vi "Diagnostic.vi"() -> ()   [LabVIEW 2015]
uses:
  Type/_GUI Method.ctl
  Type/_Lens Property.ctl
  Type/_Mass Range Property.ctl
  Type/_Mass Range Parameters.ctl
  Type/_RT Res Type.ctl
  Type/_Run Mode.ctl
  Type/_Run State.ctl
  Type/_File Type.ctl
  Type/_RT Command.ctl
  Type/_Data Operation.ctl
  Type/_Run Module.ctl
  Configuration/_Global Configuration.vi
  <vilib>/Utility/config.llb/Read Key (Path).vi
  <vilib>/Utility/config.llb/Read Key (String).vi
  <vilib>/printing/ReportDocExtensions.llb/Append Front Panel Image to Report (path).vi
  <vilib>/Utility/config.llb/Write Key (Path).vi
  <vilib>/Utility/config.llb/Write Key (String).vi
  <vilib>/Utility/miscctls.llb/LVRectTypeDef.ctl
  <vilib>/Utility/NIReport.llb/NI_report.lvclass
  <vilib>/Utility/NIReport.llb/NI_ReportGenerationCore.lvlib
  <vilib>/Utility/config.llb/NI_LVConfig.lvlib
panel:
  in  "Control 4":bool
  in  "Control 3":bool
  in  "Control 2":bool
  in  "Control 1":bool
  out "H Current 4":dbl
  out "H Current 3":dbl
  out "H Current 2":dbl
  out "H Current 1":dbl
  in  "Heater 4":dbl
  in  "Heater 3":dbl
  in  "Heater 2":dbl
  in  "Heater 1":dbl
  in  "Run Mode":T1
  in  "Q2DC EN":bool
  in  "Count1":dbl=400.0 caption="Lens Value" format="%#.3f"
  in  "Count2":dbl=400.0 caption="High Value" format="%#.3f"
  in  "Time1":dbl=1.0 caption="Low Dwell (ms)" format="%#.3f"
  in  "Time2":dbl=1.0 caption="High Dwell (ms)" format="%#.3f"
  in  "Scans":i32=1
  in  "Step Size":dbl=-1.0 format="%#.3f"
  in  "Scan Type":u8(ring) items=["Single", "Dual", "Ramp"]
  in  "Unit":bool
  in  "Q1DC EN":bool
  in  "Q1 POL":bool
  in  "Q2 POL":bool
  out "DAC Value":i32=98187
  in  "Lens Table":i32(listbox)
  in  "Swtich Polarity":bool
  in  "Run":bool
  out "Dual Run":bool
  out "Spectrum":cluster{"Mass":dbl[], "Data in cps":dbl[]}[](graph)=[{"Mass"=[664.0], "Data in cps"=[]}, {"Mass"=[800.0], "Data in cps"=[]}, {"Mass"=[700.0], "Data in cps"=[]}]
  in  "Cancel":bool
  in  "NewMethod":bool
  in  "Method Path":path
  in  "Method":T2={"Lenses"=[{"Scan Type"=0, "Scans"=1, "Time 1"=1.0, "Time 2"=1.0, "Value 1"=400.0, "Value 2"=400.0, "Step Size"=-1.0}, {"Scan Type"=0, "Scans"=1, "Time 1"=1.0, "Time 2"=1.0, "Value 1"=150.0, "Value 2"=150.0, "Step Size"=1.0}, {"Scan Type"=0, "Scans"=1, "Time 1"=1.0, "Time 2"=1.0, "Value 1"=32000.0, "Value 2"=32000.0, "Step Size"=1.0}, {"Scan Type"=0, "Scans"=1, "Time 1"=1.0, "Time 2"=1.0, "Value 1"=400.0, "Value 2"=400.0, "Step Size"=1.0}, {"Scan Type"=0, "Scans"=1, "Time 1"=1.0, "Time 2"=1.0, "Value 1"=150.0, "Value 2"=150.0, "Step Size"=1.0}, {"Scan Type"=0, "Scans"=1, "Time 1"=1.0, "Time 2"=1.0, "Value 1"=64000.0, "Value 2"=64000.0, "Step Size"=1.0}, {"Scan Type"=0, "Scans"=1, "Time 1"=1.0, "Time 2"=1.0, "Value 1"=420.0, "Value 2"=420.0, "Step Size"=1.0}, {"Scan Type"=0, "Scans"=1, "Time 1"=1.0, "Time 2"=1.0, "Value 1"=30.0, "Value 2"=30.0, "Step Size"=1.0}, {"Scan Type"=0, "Scans"=1, "Time 1"=1.0, "Time 2"=1.0, "Value 1"=15.0, "Value 2"=15.0, "Step Size"=1.0}, {"Scan Type"=0, "Scans"=1, "Time 1"=1.0, "Time 2"=1.0, "Value 1"=0.0, "Value 2"=0.0, "Step Size"=1.0}, {"Scan Type"=0, "Scans"=1, "Time 1"=1.0, "Time 2"=1.0, "Value 1"=0.0, "Value 2"=0.0, "Step Size"=1.0}, {"Scan Type"=0, "Scans"=1, "Time 1"=1.0, "Time 2"=1.0, "Value 1"=0.0, "Value 2"=0.0, "Step Size"=1.0}, {"Scan Type"=0, "Scans"=1, "Time 1"=1.0, "Time 2"=1.0, "Value 1"=0.0, "Value 2"=0.0, "Step Size"=1.0}, {"Scan Type"=0, "Scans"=1, "Time 1"=1.0, "Time 2"=1.0, "Value 1"=0.0, "Value 2"=0.0, "Step Size"=1.0}, {"Scan Type"=0, "Scans"=1, "Time 1"=1.0, "Time 2"=1.0, "Value 1"=-0.5, "Value 2"=-0.5, "Step Size"=1.0}, {"Scan Type"=0, "Scans"=1, "Time 1"=1.0, "Time 2"=1.0, "Value 1"=-2.0, "Value 2"=-2.0, "Step Size"=1.0}, {"Scan Type"=0, "Scans"=1, "Time 1"=1.0, "Time 2"=1.0, "Value 1"=-1.2, "Value 2"=-1.2, "Step Size"=1.0}, {"Scan Type"=0, "Scans"=1, "Time 1"=1.0, "Time 2"=1.0, "Value 1"=0.0, "Value 2"=0.0, "Step Size"=1.0}, {"Scan Type"=0, "Scans"=1, "Time 1"=1.0, "Time 2"=1.0, "Value 1"=-240.0, "Value 2"=-240.0, "Step Size"=1.0}, {"Scan Type"=0, "Scans"=1, "Time 1"=1.0, "Time 2"=1.0, "Value 1"=-50.0, "Value 2"=-50.0, "Step Size"=1.0}, {"Scan Type"=0, "Scans"=1, "Time 1"=1.0, "Time 2"=1.0, "Value 1"=-52.0, "Value 2"=-52.0, "Step Size"=1.0}, {"Scan Type"=0, "Scans"=1, "Time 1"=1.0, "Time 2"=1.0, "Value 1"=-100.0, "Value 2"=-100.0, "Step Size"=1.0}, {"Scan Type"=0, "Scans"=1, "Time 1"=1.0, "Time 2"=1.0, "Value 1"=-54.0, "Value 2"=-54.0, "Step Size"=1.0}, {"Scan Type"=0, "Scans"=1, "Time 1"=1.0, "Time 2"=1.0, "Value 1"=-400.0, "Value 2"=-400.0, "Step Size"=1.0}, {"Scan Type"=0, "Scans"=1, "Time 1"=1.0, "Time 2"=1.0, "Value 1"=30.0, "Value 2"=30.0, "Step Size"=1.0}, {"Scan Type"=0, "Scans"=1, "Time 1"=1.0, "Time 2"=1.0, "Value 1"=2000.0, "Value 2"=2000.0, "Step Size"=1.0}, {"Scan Type"=0, "Scans"=1, "Time 1"=1.0, "Time 2"=1.0, "Value 1"=-6000.0, "Value 2"=-6000.0, "Step Size"=1.0}, {"Scan Type"=0, "Scans"=1, "Time 1"=1.0, "Time 2"=1.0, "Value 1"=0.0, "Value 2"=0.0, "Step Size"=1.0}, {"Scan Type"=0, "Scans"=1, "Time 1"=1.0, "Time 2"=1.0, "Value 1"=0.0, "Value 2"=0.0, "Step Size"=1.0}, {"Scan Type"=0, "Scans"=1, "Time 1"=1.0, "Time 2"=1.0, "Value 1"=250.0, "Value 2"=250.0, "Step Size"=1.0}, {"Scan Type"=0, "Scans"=1, "Time 1"=1.0, "Time 2"=1.0, "Value 1"=-250.0, "Value 2"=-250.0, "Step Size"=1.0}, {"Scan Type"=0, "Scans"=1, "Time 1"=1.0, "Time 2"=1.0, "Value 1"=250.0, "Value 2"=250.0, "Step Size"=1.0}, {"Scan Type"=0, "Scans"=1, "Time 1"=1.0, "Time 2"=1.0, "Value 1"=-250.0, "Value 2"=-250.0, "Step Size"=1.0}, {"Scan Type"=0, "Scans"=1, "Time 1"=1.0, "Time 2"=1.0, "Value 1"=500.0, "Value 2"=500.0, "Step Size"=1.0}, {"Scan Type"=0, "Scans"=1, "Time 1"=1.0, "Time 2"=1.0, "Value 1"=-500.0, "Value 2"=-500.0, "Step Size"=1.0}, {"Scan Type"=0, "Scans"=1, "Time 1"=1.0, "Time 2"=1.0, "Value 1"=0.55, "Value 2"=0.55, "Step Size"=1.0}, {"Scan Type"=0, "Scans"=1, "Time 1"=1.0, "Time 2"=1.0, "Value 1"=0.0, "Value 2"=0.0, "Step Size"=1.0}, {"Scan Type"=0, "Scans"=1, "Time 1"=1.0, "Time 2"=1.0, "Value 1"=100.0, "Value 2"=100.0, "Step Size"=1.0}, {"Scan Type"=0, "Scans"=1, "Time 1"=1.0, "Time 2"=1.0, "Value 1"=0.0, "Value 2"=0.0, "Step Size"=1.0}, {"Scan Type"=0, "Scans"=1, "Time 1"=1.0, "Time 2"=1.0, "Value 1"=5.0, "Value 2"=5.0, "Step Size"=1.0}, {"Scan Type"=0, "Scans"=1, "Time 1"=1.0, "Time 2"=1.0, "Value 1"=0.0, "Value 2"=0.0, "Step Size"=1.0}, {"Scan Type"=0, "Scans"=1, "Time 1"=1.0, "Time 2"=1.0, "Value 1"=0.0, "Value 2"=0.0, "Step Size"=1.0}, {"Scan Type"=0, "Scans"=1, "Time 1"=1.0, "Time 2"=1.0, "Value 1"=100.0, "Value 2"=100.0, "Step Size"=1.0}, {"Scan Type"=0, "Scans"=1, "Time 1"=1.0, "Time 2"=1.0, "Value 1"=0.0, "Value 2"=0.0, "Step Size"=1.0}, {"Scan Type"=0, "Scans"=1, "Time 1"=1.0, "Time 2"=1.0, "Value 1"=5.0, "Value 2"=5.0, "Step Size"=1.0}, {"Scan Type"=0, "Scans"=1, "Time 1"=1.0, "Time 2"=1.0, "Value 1"=5000.0, "Value 2"=5000.0, "Step Size"=1.0}, {"Scan Type"=0, "Scans"=1, "Time 1"=1.0, "Time 2"=1.0, "Value 1"=0.0, "Value 2"=0.0, "Step Size"=1.0}, {"Scan Type"=0, "Scans"=1, "Time 1"=1.0, "Time 2"=1.0, "Value 1"=100.0, "Value 2"=100.0, "Step Size"=1.0}, {"Scan Type"=0, "Scans"=1, "Time 1"=1.0, "Time 2"=1.0, "Value 1"=0.0, "Value 2"=0.0, "Step Size"=1.0}, {"Scan Type"=0, "Scans"=1, "Time 1"=1.0, "Time 2"=1.0, "Value 1"=5.0, "Value 2"=5.0, "Step Size"=1.0}, {"Scan Type"=0, "Scans"=1, "Time 1"=1.0, "Time 2"=1.0, "Value 1"=1000.0, "Value 2"=1000.0, "Step Size"=1.0}, {"Scan Type"=0, "Scans"=1, "Time 1"=1.0, "Time 2"=1.0, "Value 1"=1.0, "Value 2"=1.0, "Step Size"=1.0}], "Mass Ranges"=[], "Acquire"=FALSE, "MCA"=FALSE, "Q1DC EN"=FALSE, "Q1 POL"=FALSE, "Q3 POL"=FALSE, "Q1 RF  EN"=FALSE, "Averaging"=FALSE, "Log Scale"=FALSE, "CPS"=FALSE, "Unit"=FALSE, "Data Path"=path "", "Run Mode"=enum."MRM (Q1/Q2)", "Fixed Mass (amu)"=0.0, "Q3DC EN"=FALSE, "Q3 RF  EN"=FALSE, "Negative"=FALSE} {"Mass Ranges"."Res" items=["High/High", "Medium/Medium", "Low/Low", "High/Medium", "High/Low", "Medium/High", "Medium/Low", "Low/High", "Low/Medium"]}
  out "Run Time":i32 caption="Run Time (ms)"
  in  "Log Scale":bool
  in  "Scan#":u32=1 caption="Current Scan #"
  in  "CPS":bool
  in  "Averaging":bool
  in  "MCA":bool
  in  "Acquire":bool
  in  "BloUpdate":bool
  out "Data File:":path=path "C:/Users/Min/Projects/Sniffer"
  # "Selected Lens Property"
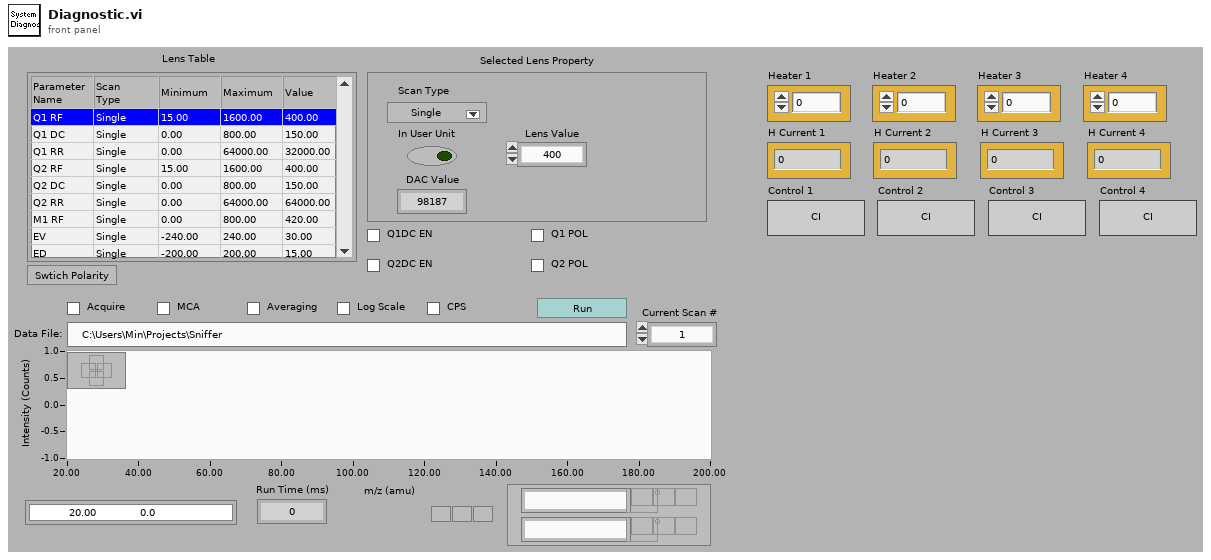
[diagram p1: front panel]
types:
  T1 = typedef "_Run Mode.ctl" = enum16{"MRM (Q1/Q2)", "Q1 Scan", "Q1 SRM", "Q2 Scan", "Q2 SRM", "Product Scan", "Precursor Scan", "Neutral Loss", "Neutral Gain"}
  T2 = typedef "_GUI Method.ctl" = cluster{"Lenses":T3[], "Mass Ranges":T4[], "Acquire":bool, "MCA":bool, "Q1DC EN":bool, "Q1 POL":bool, "Q3 POL":bool, "Q1 RF  EN":bool, "Averaging":bool, "Log Scale":bool, "CPS":bool, "Unit":bool, "Data Path":path, "Run Mode":T1, "Fixed Mass (amu)":dbl, "Q3DC EN":bool, "Q3 RF  EN":bool, "Negative":bool}
  T3 = typedef "_Lens Property.ctl" = cluster{"Scan Type":u8, "Scans":i32, "Time 1":dbl, "Time 2":dbl, "Value 1":dbl, "Value 2":dbl, "Step Size":dbl}
  T4 = typedef "_Mass Range Property.ctl" = cluster{"Start":dbl, "Stop":dbl, "Step Size":dbl, "Steps":i32, "Dwell":dbl, "Parameters":T5[], "Res":T6}
  T5 = typedef "_Mass Range Parameters.ctl" = cluster{"Name":string, "Ch#":u8, "StartV":dbl, "StopV":dbl, "StepV":dbl, "Index":u8}
  T6 = typedef "_RT Res Type.ctl" = u16
  T7 = typedef "_Run State.ctl" = enum16{"Init", "Update", "Start", "End", "Error"}
  T8 = typedef "_RT Instrument 2.ctl" = cluster{"Table":T9[], "Instrument":string[]}
  T9 = typedef "_RT Configuration 2.ctl" = cluster{"Name":string, "Ch#":u8, "Min":dbl, "Max":dbl, "Def+":dbl, "Def-":dbl, "Offset":dbl, "Slope":dbl, "Type":u8, "Description":string, "SettleT":dbl}
  T10 = typedef "_File Type.ctl" = enum16{"Configuration", "Old Configuration", "Calibration", "Resolution", "Diagnostic Method", "Old Method", "Acq Method", "Samp List"}
  T11 = typedef "LVRectTypeDef.ctl" = cluster{"Left":i16, "Top":i16, "Right":i16, "Bottom":i16}
  T12 = enum16{"Standard Report", "HTML", "Word", "Excel"}
  T13 = typedef "_RT Command.ctl" = enum16{"xml Start Run", "xml Start Actual Run", "xml Stop Run", "xml Runtime Update", "xml Get Status", "xml Get Table", "xml Set Table", "xml Get Configuration", "xml System Status", "xml Set LC Input Logic", "xml Get Data", "xml Get Info", "Start", "StartActualRun", "Stop", "Runtime Update", "Get Data", "Get Info", "Get Status", "Get Param", "Get Config", "Get Table", "Read ADC", "Set Oscillator", "Update Config", "Update Table", "Set All Pol", "Set Pol and DC", "Set Max Mass", "Toggle RP", "Toggle EL", "Set PIC", "Initialize Turbo", "Send Turbo Comm", "Close Turbo", "P1", "P2", "P3", "Send Serial", "Set LC Out", "Get LC In", "Read VAC", "Test Table", "Toggle Power", "Get Startup", "Set Startup", "Get ADC Table", "Set ADC Table", "Get Brief Status", "Get Detail Status", "Auxiliary Update", "Set CC Logics", "Set CC Input Logics", "Ignore Error", "invalid"}
  T14 = typedef "_Data Operation.ctl" = enum8{"Initialize", "Get Data", "Set Data", "Close"}
  T15 = enum32{"Bad", "Idle", "Run top level", "Running"}
  T16 = typedef "NI_LVConfig.lvlib/Config Data RefNum.ctl" = refnum<k1>
  T17 = cluster{"Method":T2, "Update":bool, "Running":bool, "Method Path":path}
  T18 = typedef "_Current Data.ctl" = cluster{"Scan#":i32, "Run Time (mS)":i32, "TIC X":dbl[], "TIC Y":dbl[][], "MassRange":cluster{"X Title":string, "X":dbl[], "Y":i32[]}[], "Fixed Mass (amu)":dbl, "Method":T19}
  T19 = typedef "_XML Expt.ctl" = cluster{"StartT(mS)":i32, "#Cycles":i32, "PauseT(uS)":i32, "ScanType":i32, "Polarity":u8, "FixedMass":dbl, "DelayT(mS)":i32, "Active Ch":T20[], "Mass Range":T4[]}
  T20 = typedef "_XML Lens.ctl" = cluster{"Value":dbl, "ChID":u8}
  T21 = cluster{"Scan Type":u8, "Unit":bool, "Count1":dbl, "Count2":dbl, "Time1":dbl, "Time2":dbl, "Scans":i32, "Step Size":dbl, "Lens Table":i32}
  T22 = cluster{"Scan Type":u8, "Unit":bool, "Count1":dbl, "Count2":dbl, "Time1":dbl, "Time2":dbl, "Scans":i32, "Step Size":dbl, "Start DAC":i32, "Ramp Time (ms)":i32}
  T23 = cluster{bool, "Value 1":dbl, "Value 2":dbl, "Step Size":dbl}
  T24 = typedef "_Run Module.ctl" = u16
  T25 = cluster{"NewVal":bool, "Count1":dbl, "Count2":dbl, "Step Size":dbl}
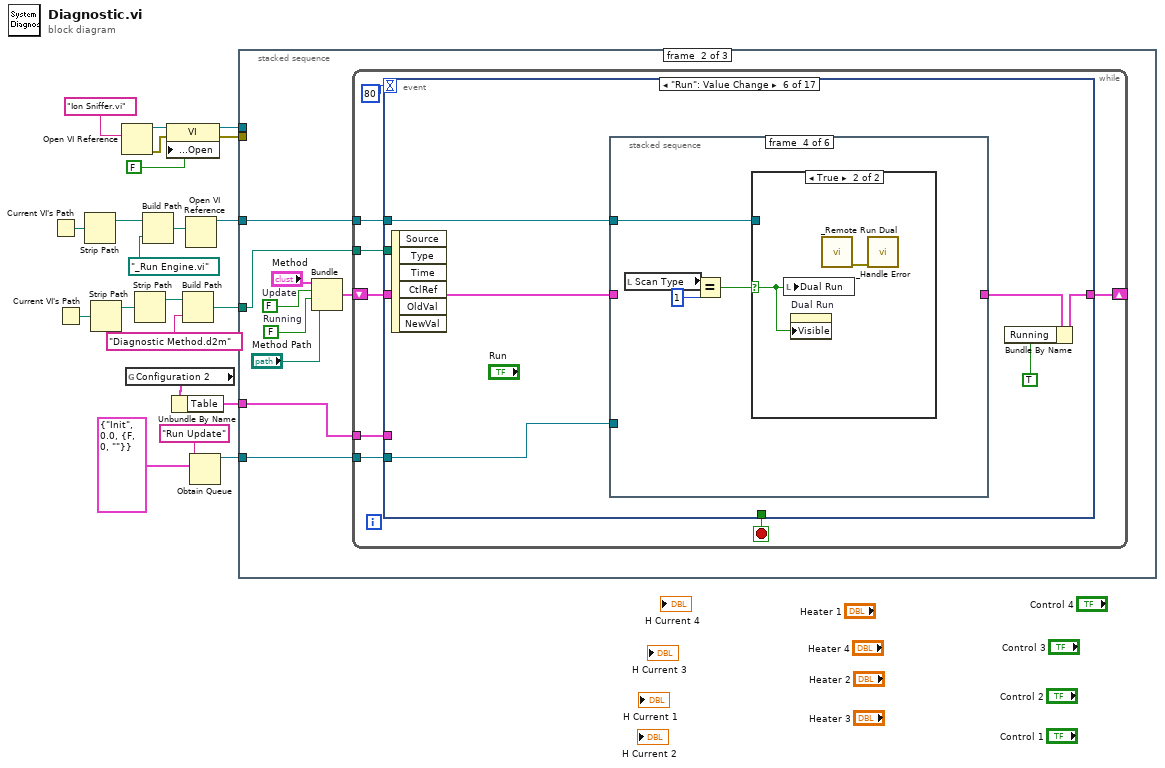
[diagram p0: block diagram]
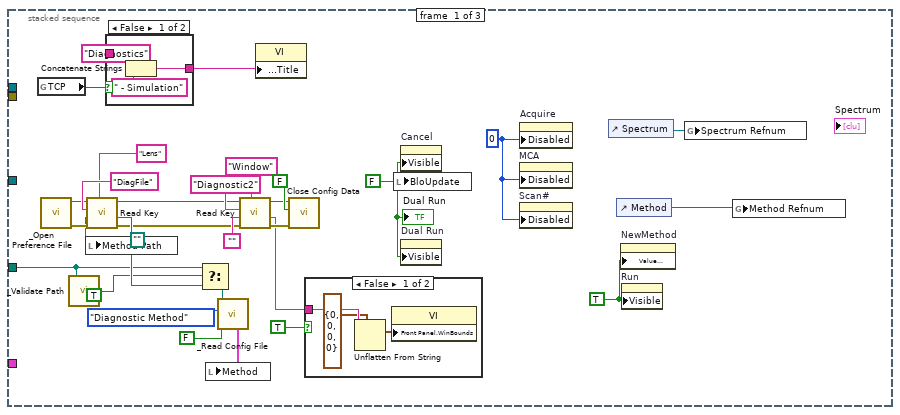
[diagram p2: hidden frame]
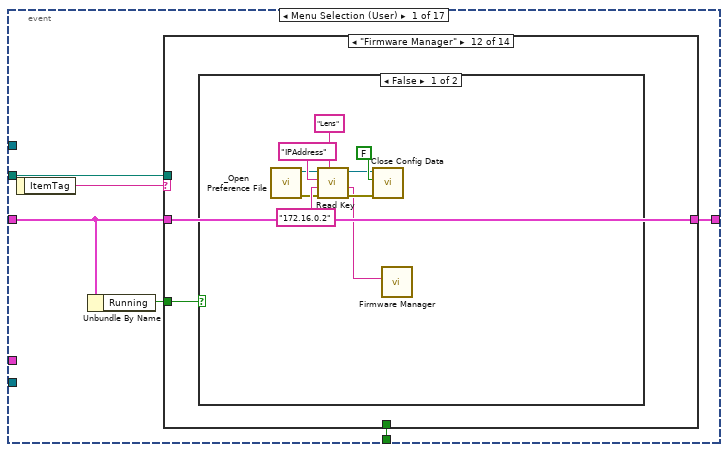
[diagram p5: hidden frame]
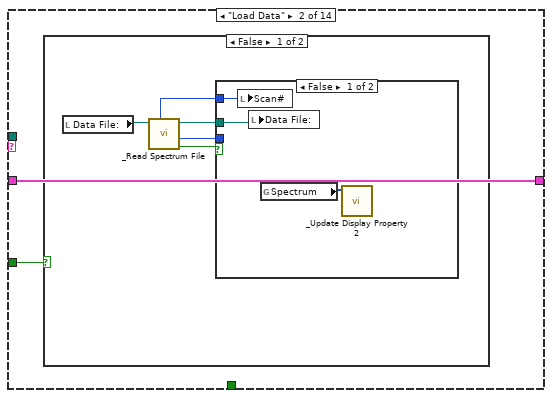
[diagram p7: hidden frame]
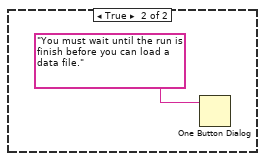
[diagram p9: hidden frame]
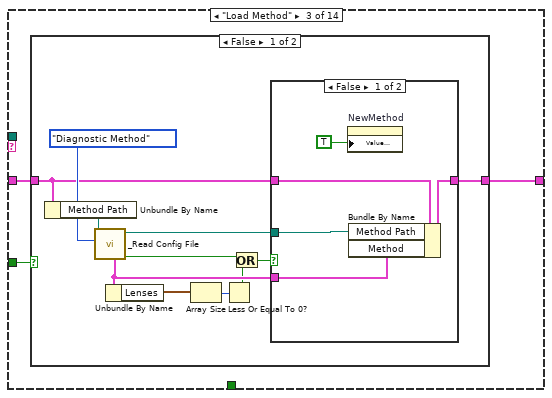
[diagram p10: hidden frame]
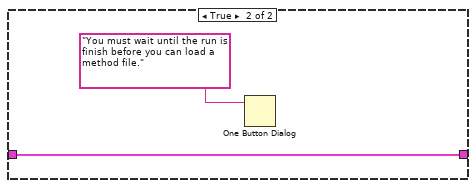
[diagram p12: hidden frame]
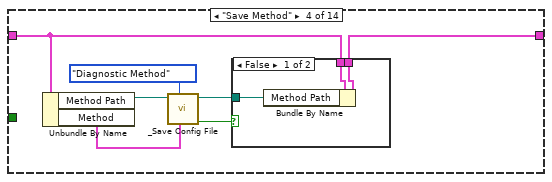
[diagram p13: hidden frame]
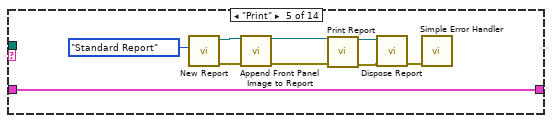
[diagram p15: hidden frame]
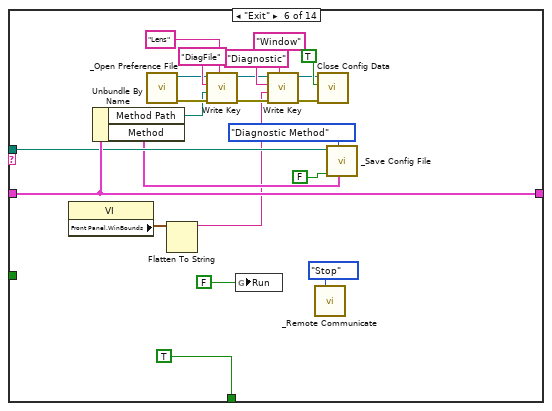
[diagram p16: hidden frame]
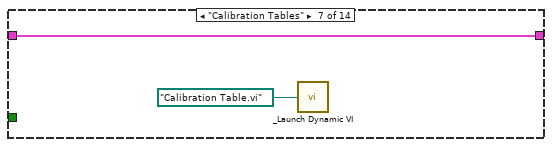
[diagram p17: hidden frame]
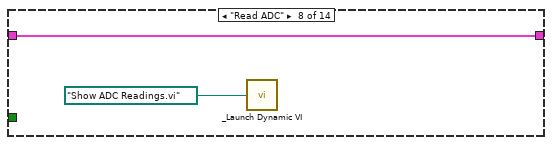
[diagram p18: hidden frame]
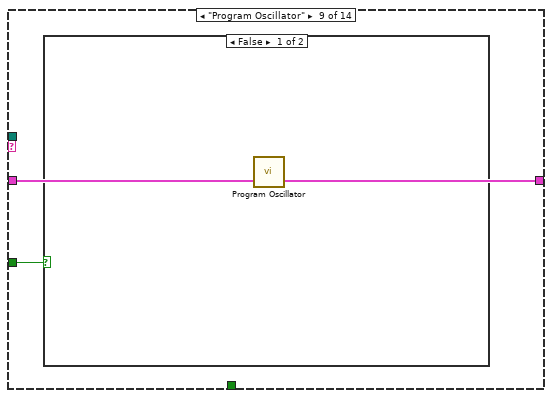
[diagram p19: hidden frame]
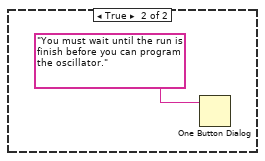
[diagram p20: hidden frame]
diagram:
  n1 = Current VI's Path() -> (path=w18:path)
  n2 = Current VI's Path() -> (path=w8:path)
  n3 = Strip Path(path=w18) -> (stripped path=w14:path)  [unwired: 1 out]
  n4 = Strip Path(path=w8) -> (stripped path=w9:path)  [unwired: 1 out]
  n5 = Open VI Reference(vi path="Ion Sniffer.vi") -> (vi reference=w5:refnum<vi>, error out=w4:errorcluster)  [unwired: 1 in, 4 out]
  n6 = global read "_Global Configuration.vi" "Configuration 2"() -> (w13:T8)
  n7 = Strip Path(path=w9) -> (stripped path=w10:path)  [unwired: 1 out]
  n8 = Build Path(base path=w14, name or relative path=path "_Run Engine.vi") -> (appended path=w16:path)
  n9 = property class="VI"(reference=w5, error in=w4, "Front Panel Window:Open"=FALSE) -> (reference out=w2:refnum<vi>, error out=w1:errorcluster)
  n10 = Unbundle By Name(w13) -> ("Table"=w12:T9[])
  n11 = Build Path(base path=w10, name or relative path="Diagnostic Method.d2m") -> (appended path=w7:path)
  n12 = Open VI Reference(vi path=w16) -> (vi reference=w15:refnum<vi>)  [unwired: 1 in, 5 out]
  n13 = Obtain Queue(name (unnamed)="Run Update", element data type=cluster{T7, dbl, "error out":errorcluster} {enum."Init", 0.0, "error out"={"status"=FALSE, "code"=0, "source"=""}}) -> (queue out=w19:refnum<queue>)  [unwired: 3 in, 2 out]
  n14 = stacked-sequence {
    tunnel: w19 -> [_ w68 w630]
    tunnel: w15 -> [_ w67 w629]
    tunnel: w12 -> [_ w61 _]
    tunnel: w7 -> [w24 w60 _]
    tunnel: w2 -> [_ _ w625]
    tunnel: w1 -> [_ _ w624]
    frame #0 {
      w28 = TRUE ("Visible")
      w49 = u8 0 ("Disabled")
      w42 = FALSE ("Unit")
      n15 = global read "_Global Configuration.vi" "TCP"() -> (w50:bool)
      n16 = call "_Open Preference File.vi"() -> ("error"=w45:errorcluster, "refnum"=w46:T16)  [unwired: 3 in, 3 out]
      n17 = call "_Validate Path.vi"("Check Exist (F)"=TRUE, "path"=w24) -> ("Valid"=w25:bool)  [unwired: 2 in]
      n18 = call-poly <vilib>:"Read Key.vi"("section"="Lens", "error in (no error)"=w45, "default value"=path "", "key"="DiagFile", "refnum"=w46) -> ("error out"=w32:errorcluster, "value"=w38:path, "refnum out"=w33:T16)  [unwired: 4 out]
      n19 = local write "Method Path"(w38) -> ()
      n20 = case shown="False" w50 {
        tunnel: "Diagnostics" ("string") -> [w58 w59]
        tunnel: [w56 w59] -> w51
        frame False {
          n21 = Concatenate Strings(w58, " - Simulation" ("string")) -> (w56:string)
        }
        frame True {
        }
      }
      n22 = Select(t=w24, s=w25, f=w38) -> (s? t:f=w37:path)
      n23 = call "_Read Config File.vi"("advisory dialog? (display:T)"=FALSE, "File Type (config)"=_File_Type."Diagnostic Method", "start path  (Not A Path)"=w37) -> ("GUI Method"=w40:T2)  [unwired: 8 out]
      n24 = local write "Method"(w40) -> ()
      n25 = call-poly <vilib>:"Read Key.vi"("section"="Window", "error in (no error)"=w32, "default value"="", "key"="Diagnostic2" ("section"), "refnum"=w33) -> ("error out"=w30:errorcluster, "value"=w29:string, "refnum out"=w31:T16)  [unwired: 1 in, 3 out]
      n26 = property class="VI"("Front Panel Window:Title"=w51) -> ()  [unwired: 2 in, 2 out]
      n27 = call <vilib>:"Close Config Data.vi"("error in (no error)"=w30, "write file if changed (T)"=FALSE ("write configuration file? (F)"), "refnum"=w31) -> ()  [unwired: 9 out]
      n28 = case shown="False" TRUE {
        tunnel: w29 -> [w55 _]
        frame False {
          n29 = Unflatten From String(type=T11 {"Left"=0, "Top"=0, "Right"=0, "Bottom"=0} ("Front Panel Window:Window Bounds"), binary string=w55) -> (value=w53:T11)  [unwired: 1 in, 4 out]
          n30 = property class="VI"("Front Panel.WinBounds"=w53) -> ()  [unwired: 2 in, 2 out]
        }
        frame True {
        }
      }
      n31 = local write "BloUpdate"(w42) -> ()
      n32 = property on="Cancel" class="Bool"("Visible"=w42) -> ()  [unwired: 2 in, 2 out]
      n33 = property on="Dual Run" class="Bool (strict)"("Visible"=w42) -> ()  [unwired: 2 in, 2 out]
      n34 = property on="Acquire" class="Bool (strict)"("Disabled"=w49) -> ()  [unwired: 2 in, 2 out]
      n35 = property on="MCA" class="Bool (strict)"("Disabled"=w49) -> ()  [unwired: 2 in, 2 out]
      n36 = property on="Scan#" class="DigNum (strict)"("Disabled"=w49) -> ()  [unwired: 2 in, 2 out]
      n37 = control-ref of="Spectrum"() -> (w27:refnum<vi>)
      n38 = control-ref of="Method"() -> (w26:refnum<vi>)
      n39 = property on="NewMethod" class="Bool (strict)"("Value (Signaling)"=w28) -> ()  [unwired: 2 in, 2 out]
      n40 = property on="Run" class="Bool"("Visible"=w28) -> ()  [unwired: 2 in, 2 out]
      n41 = global write "_Global Configuration.vi" "Spectrum Refnum"(w27) -> ()
      n42 = global write "_Global Configuration.vi" "Method Refnum"(w26) -> ()
      "Dual Run" <- w42
    }
    frame #1 {
      w64 = FALSE  # Running
      w65 = FALSE  # Update
      n43 = Bundle("Method"="Method", "Update"=w65, "Running"=w64, "Method Path"="Method Path") -> (w63:T17)  [unwired: 1 out]
      n44 = while {
        shift-right: [w73] -> _
        shift-left: w63 -> [w75]
        tunnel: w68 -> [w72]
        tunnel: w67 -> [w71]
        tunnel: w61 -> [w70]
        tunnel: w60 -> [w69]
        stop <- w76 stop-if-true
        n45 = event shown="[5] \"Run\": Value Change" {
          selector: _ -> [_ _ _ _ _ _ _ _ _ _ _ _ _ _ _ _ _]
          dyn-events: _ -> [_ _ _ _ _ _ _ _ _ _ _ _ _ _ _ _ _]
          timeout: 80 -> [_ _ _ _ _ _ _ _ _ _ _ _ _ _ _ _ _]
          tunnel: [w80 w259 _ _ _ _ _ _ _ _ _ _ _ _ _ _ _] -> w76
          tunnel: w75 -> [w79 w251 w262 w338 w382 w412 w447 w469 w482 w536 w552 w572 w586 w588 w605 w609 w623]
          tunnel: [w81 w251 w264 w338 w381 w409 w446 w469 w481 w537 w565 w571 w582 w588 w604 w608 w621] -> w73
          tunnel: w72 -> [_ _ w263 _ _ w413 _ _ _ _ _ _ _ _ _ _ _]
          tunnel: w71 -> [_ _ _ _ _ w414 w445 _ _ _ _ _ _ _ _ _ _]
          tunnel: w70 -> [_ _ _ w335 _ _ _ _ w485 _ _ _ _ _ _ w613 _]
          tunnel: w69 -> [w77 w248 _ _ _ _ _ _ _ _ _ _ _ _ _ _ _]
          event Menu Selection (User) {
            n46 = event-data() -> ("ItemTag"=w82:string)  [unwired: 1 out]
            n47 = Unbundle By Name(w79) -> ("Running"=w78:bool)
            n48 = case shown="\"Firmware Manager\"" w82 {
              tunnel: w78 -> [_ w85 w97 _ _ _ _ _ w164 w167 w211 w225 _ _]
              tunnel: w79 -> [w83 w84 w96 w118 w130 w152 w159 w161 w163 w166 w210 w224 w236 w237]
              tunnel: [w83 w84 w95 w117 w130 w152 w159 w161 w163 w166 w210 w224 w236 w237] -> w81
              tunnel: [_ _ _ _ _ TRUE _ _ _ _ _ _ _ _] -> w80
              tunnel: w77 -> [_ _ _ _ _ w146 _ _ _ _ _ _ _ _]
              frame Default {
              }
              frame "Load Data" {
                n49 = case shown="False" w85 {
                  frame False {
                    n50 = local read "Data File:"() -> (w88:path)
                    n51 = call "_Read Spectrum File.vi"("start path  (Not A Path)"=w88) -> ("error"=w90:bool, "TIC"=w89:u32, "new file path"=w87:path, "Scan# out"=w86:u32)  [unwired: 2 in, 3 out]
                    n52 = case shown="False" w90 {
                      tunnel: w89 -> [_ _]
                      tunnel: w87 -> [w93 _]
                      tunnel: w86 -> [w92 _]
                      frame False {
                        n53 = local write "Scan#"(w92) -> ()
                        n54 = local write "Data File:"(w93) -> ()
                        n55 = global read "_Global Configuration.vi" "Spectrum"() -> (w91:i32[])
                        n56 = call "_Update Display Property 2.vi"("Spectrum in"=w91) -> ()  [unwired: 7 out]
                      }
                      frame True {
                      }
                    }
                  }
                  frame True {
                    n57 = One Button Dialog(message="You must wait until the run is finish before you can load a data file.") -> ()  [unwired: 2 out]
                  }
                }
              }
              frame "Load Method" {
                n58 = case shown="False" w97 {
                  tunnel: w96 -> [w106 w115]
                  tunnel: [w98 w115] -> w95
                  frame False {
                    n59 = Unbundle By Name(w106) -> ("Method Path"=w108:path)
                    n60 = call "_Read Config File.vi"("File Type (config)"=_File_Type."Diagnostic Method", "start path  (Not A Path)"=w108) -> ("error"=w101:bool, "new file path"=w105:path, "GUI Method"=w104:T2)  [unwired: 1 in, 6 out]
                    n61 = Unbundle By Name(w104) -> ("Lenses"=w103:T3[])
                    n62 = Array Size(array=w103) -> (size(s)=w102:i32)
                    n63 = Less Or Equal To 0?(x=w102) -> (x <= 0?=w100:bool)
                    n64 = Or(x=w101, y=w100) -> (x .or. y?=w99:bool)
                    n65 = case shown="False" w99 {
                      tunnel: w106 -> [w113 w114]
                      tunnel: w104 -> [w110 _]
                      tunnel: w105 -> [w111 _]
                      tunnel: [w112 w114] -> w98
                      frame False {
                        n66 = property on="NewMethod" class="Bool (strict)"("Value (Signaling)"=TRUE) -> ()  [unwired: 2 in, 2 out]
                        n67 = Bundle By Name(cluster=w113, "Method Path"=w111, "Method"=w110) -> (w112:T17)
                      }
                      frame True {
                      }
                    }
                  }
                  frame True {
                    n68 = One Button Dialog(message="You must wait until the run is finish before you can load a method file.") -> ()  [unwired: 2 out]
                  }
                }
              }
              frame "Save Method" {
                n69 = Unbundle By Name(w118) -> ("Method Path"=w121:path, "Method"=w119:T2)
                n70 = call "_Save Config File.vi"("GUI Method"=w119, "File Type (config)"=_File_Type."Diagnostic Method", "start path  (Not A Path)"=w121) -> ("error"=w122:bool, "new file path"=w123:path)  [unwired: 5 in, 2 out]
                n71 = case shown="False" w122 {
                  tunnel: w123 -> [w125 _]
                  tunnel: w118 -> [w126 w127]
                  tunnel: [w124 w127] -> w117
                  frame False {
                    n72 = Bundle By Name(cluster=w126, "Method Path"=w125) -> (w124:T17)
                  }
                  frame True {
                  }
                }
              }
              frame "Print" {
                n73 = call <vilib>:"New Report.vi"("report type"=T12."Standard Report") -> ("report out"=w134:refnum<class "NI_report.lvclass">, "error out"=w133:errorcluster)  [unwired: 5 in, 8 out]
                n74 = call-poly <vilib>:"Append Front Panel Image to Report.vi"("report in"=w134, "error in (no error)"=w133) -> ("report out"=w132:refnum<class "NI_report.lvclass">, "error out"=w131:errorcluster)  [unwired: 6 in, 6 out]
                n75 = call-dynamic "Print Report.vi"("report in"=w132, "error in (no error)"=w131) -> ("report out"=w136:refnum<class "NI_report.lvclass">, "error out"=w135:errorcluster)  [unwired: 2 in, 10 out]
                n76 = call-dynamic "Dispose Report.vi"("report in"=w136, "error in (no error)"=w135) -> ("error out"=w129:errorcluster)  [unwired: 3 in, 10 out]
                n77 = call <vilib>:"Simple Error Handler.vi"("error in (no error)"=w129) -> ()  [unwired: 1 in, 8 out]
              }
              frame "Exit" {
                n78 = property class="VI"() -> ("Front Panel.WinBounds"=w138:T11)  [unwired: 2 in, 2 out]
                n79 = Unbundle By Name(w152) -> ("Method Path"=w153:path, "Method"=w145:T2)
                n80 = call "_Open Preference File.vi"() -> ("error"=w154:errorcluster, "refnum"=w155:T16)  [unwired: 3 in, 3 out]
                n81 = Flatten To String(anything=w138) -> (data string=w137:string)  [unwired: 1 in, 4 out]
                n82 = call-poly <vilib>:"Write Key.vi"("section"="Lens", "error in (no error)"=w154, "value"=w153, "key"="DiagFile", "refnum"=w155) -> ("error out"=w140:errorcluster, "refnum out"=w142:T16)  [unwired: 5 out]
                n83 = global write "_Global Configuration.vi" "Run"(FALSE ("Update")) -> ()
                n84 = call-poly <vilib>:"Write Key.vi"("section"="Window", "error in (no error)"=w140, "value"=w137, "key"="Diagnostic" ("section"), "refnum"=w142) -> ("error out"=w139:errorcluster, "refnum out"=w141:T16)  [unwired: 1 in, 4 out]
                n85 = call "_Remote Communicate.vi"("Command"=_RT_Command."Stop") -> ()  [unwired: 5 in, 4 out]
                n86 = call <vilib>:"Close Config Data.vi"("error in (no error)"=w139, "write file if changed (T)"=TRUE ("write configuration file? (F)"), "refnum"=w141) -> ()  [unwired: 9 out]
                n87 = call "_Save Config File.vi"("GUI Method"=w145, "File Type (config)"=_File_Type."Diagnostic Method", "advisory dialog? (display:T)"=FALSE, "start path  (Not A Path)"=w146) -> ()  [unwired: 4 in, 4 out]
              }
              frame "Calibration Tables" {
                n88 = call "_Launch Dynamic VI.vi"("VI Name"=path "Calibration Table.vi" ("name or relative path")) -> ()  [unwired: 4 out]
              }
              frame "Read ADC" {
                n89 = call "_Launch Dynamic VI.vi"("VI Name"=path "Show ADC Readings.vi" ("name or relative path")) -> ()  [unwired: 4 out]
              }
              frame "Program Oscillator" {
                n90 = case shown="False" w164 {
                  frame False {
                    n91 = call "Program Oscillator.vi"() -> ()  [unwired: 1 out]
                  }
                  frame True {
                    n92 = One Button Dialog(message="You must wait until the run is finish before you can program the oscillator.") -> ()  [unwired: 2 out]
                  }
                }
              }
              frame "Load Oscillators" {
                n93 = case shown="False" w167 {
                  frame False {
                    w174 = ""
                    w180 = "Oscillator" ("section")
                    n94 = call "_Open Preference File.vi"() -> ("refnum"=w183:T16)  [unwired: 3 in, 4 out]
                    n95 = call-poly <vilib>:"Read Key.vi"("section"=w180, "default value"=w174, "key"="0" ("section"), "refnum"=w183) -> ("value"=w175:string, "refnum out"=w182:T16)  [unwired: 2 in, 4 out]
                    n96 = call-poly <vilib>:"Read Key.vi"("section"=w180, "default value"=w174, "key"="1" ("section"), "refnum"=w182) -> ("value"=w173:string, "refnum out"=w181:T16)  [unwired: 2 in, 4 out]
                    n97 = call-poly <vilib>:"Read Key.vi"("section"=w180, "default value"=w174, "key"="2" ("section"), "refnum"=w181) -> ("value"=w172:string, "refnum out"=w176:T16)  [unwired: 2 in, 4 out]
                    n98 = stacked-sequence {
                      tunnel: w175 -> [w186 _ _]
                      tunnel: [w185 _ _] -> w171
                      tunnel: w173 -> [_ w194 _]
                      tunnel: w172 -> [_ _ w202]
                      tunnel: [_ w193 _] -> w170
                      tunnel: [_ _ w201] -> w169
                      frame #0 {
                        n99 = Empty String/Path?(string/path=w186) -> (empty?=w187:bool)
                        n100 = case shown="False" w187 {
                          tunnel: w186 -> [w189 _]
                          tunnel: [w188 w192] -> w185
                          frame False {
                            n101 = call "_Remote Communicate.vi"("String"=w189, "Command"=_RT_Command."Set Oscillator") -> ("error out"=w188:errorcluster)  [unwired: 4 in, 3 out]
                          }
                          frame True {
                            n102 = call "_Construct Error Cluster.vi"("reason"="Q1-FREQ has not been programmed.") -> ("error out"=w192:errorcluster)  [unwired: 3 in, 3 out]
                          }
                        }
                      }
                      frame #1 {
                        n103 = Empty String/Path?(string/path=w194) -> (empty?=w195:bool)
                        n104 = case shown="False" w195 {
                          tunnel: w194 -> [w197 _]
                          tunnel: [w196 w200] -> w193
                          frame False {
                            n105 = call "_Remote Communicate.vi"("String"=w197, "Command"=_RT_Command."Set Oscillator") -> ("error out"=w196:errorcluster)  [unwired: 4 in, 3 out]
                          }
                          frame True {
                            n106 = call "_Construct Error Cluster.vi"("reason"="Q3-FREQ has not been programmed.") -> ("error out"=w200:errorcluster)  [unwired: 3 in, 3 out]
                          }
                        }
                      }
                      frame #2 {
                        n107 = Empty String/Path?(string/path=w202) -> (empty?=w203:bool)
                        n108 = case shown="False" w203 {
                          tunnel: w202 -> [w205 _]
                          tunnel: [w204 w208] -> w201
                          frame False {
                            n109 = call "_Remote Communicate.vi"("String"=w205, "Command"=_RT_Command."Set Oscillator") -> ("error out"=w204:errorcluster)  [unwired: 4 in, 3 out]
                          }
                          frame True {
                            n110 = call "_Construct Error Cluster.vi"("reason"="MP1-FREQ has not been programmed.") -> ("error out"=w208:errorcluster)  [unwired: 3 in, 3 out]
                          }
                        }
                      }
                    }
                    n111 = call <vilib>:"Close Config Data.vi"("write file if changed (T)"=FALSE ("write configuration file? (T)"), "refnum"=w176) -> ()  [unwired: 1 in, 9 out]
                    n112 = Merge Errors(w171, w170, w169) -> (w168:errorcluster)
                    n113 = call "_Handle Error.vi"("error in (no error)"=w168) -> ()  [unwired: 2 in, 5 out]
                  }
                  frame True {
                    n114 = One Button Dialog(message="You must wait until the run is finish before you can load the oscillators.") -> ()  [unwired: 2 out]
                  }
                }
              }
              frame "Firmware Reboot" {
                n115 = case shown="False" w211 {
                  frame False {
                    n116 = Two Button Dialog(message="You will have to wait up to 3 min for the firmware to finish rebooting.  Proceed? ") -> (T button?=w212:bool)  [unwired: 2 out]
                    n117 = case shown="True" w212 {
                      frame False {
                      }
                      frame True {
                        n118 = call "_Open Preference File.vi"() -> ("error"=w215:errorcluster, "refnum"=w216:T16)  [unwired: 3 in, 3 out]
                        n119 = call-poly <vilib>:"Read Key.vi"("section"="Lens", "error in (no error)"=w215, "default value"="172.16.0.2", "key"="IPAddress", "refnum"=w216) -> ("error out"=w217:errorcluster, "value"=w214:string, "refnum out"=w218:T16)  [unwired: 1 in, 3 out]
                        n120 = call "_Remote Reboot.vi"("IP Address"=w214) -> ()  [unwired: 2 out]
                        n121 = call <vilib>:"Close Config Data.vi"("error in (no error)"=w217, "write file if changed (T)"=FALSE ("write configuration file? (F)"), "refnum"=w218) -> ()  [unwired: 9 out]
                      }
                    }
                  }
                  frame True {
                    n122 = One Button Dialog(message="You must wait until the run is finish before you can reboot the firware.") -> ()  [unwired: 2 out]
                  }
                }
              }
              frame "Firmware Manager" {
                n123 = case shown="False" w225 {
                  frame False {
                    n124 = call "_Open Preference File.vi"() -> ("error"=w227:errorcluster, "refnum"=w228:T16)  [unwired: 3 in, 3 out]
                    n125 = call-poly <vilib>:"Read Key.vi"("section"="Lens", "error in (no error)"=w227, "default value"="172.16.0.2", "key"="IPAddress", "refnum"=w228) -> ("error out"=w229:errorcluster, "value"=w226:string, "refnum out"=w230:T16)  [unwired: 1 in, 3 out]
                    n126 = call <vilib>:"Close Config Data.vi"("error in (no error)"=w229, "write file if changed (T)"=FALSE ("write configuration file? (F)"), "refnum"=w230) -> ()  [unwired: 9 out]
                    n127 = call "Firmware Manager.vi"("cRIO IP Address"=w226) -> ()  [unwired: 2 in, 5 out]
                  }
                  frame True {
                    n128 = One Button Dialog(message="You must wait until the run is finish before you can backup or update the firware.") -> ()  [unwired: 2 out]
                  }
                }
              }
              frame "Read FPGA Map" {
                n129 = call "Show FPGA Map.vi"() -> ()  [unwired: 12 out]
              }
              frame "About" {
                n130 = call "About Box.vi"() -> ()  [unwired: 1 out]
              }
            }
          }
          event Panel Close? {
            w259 = TRUE ("Discard?")
            n131 = event-data() -> ()  [unwired: 4 out]
            n132 = property class="VI"() -> ("Front Panel.WinBounds"=w239:T11)  [unwired: 2 in, 2 out]
            n133 = Unbundle By Name(w251) -> ("Method Path"=w250:path, "Method"=w247:T2)
            n134 = call "_Remote Communicate.vi"("Command"=_RT_Command."Stop") -> ()  [unwired: 5 in, 4 out]
            n135 = Flatten To String(anything=w239) -> (data string=w238:string)  [unwired: 1 in, 4 out]
            n136 = call "_Open Preference File.vi"() -> ("error"=w254:errorcluster, "refnum"=w255:T16)  [unwired: 3 in, 3 out]
            n137 = call-poly <vilib>:"Write Key.vi"("section"="Lens", "error in (no error)"=w254, "value"=w250, "key"="DiagFile", "refnum"=w255) -> ("error out"=w242:errorcluster, "refnum out"=w243:T16)  [unwired: 5 out]
            n138 = call-poly <vilib>:"Write Key.vi"("section"="Window", "error in (no error)"=w242, "value"=w238, "key"="Diagnostic2" ("section"), "refnum"=w243) -> ("error out"=w240:errorcluster, "refnum out"=w241:T16)  [unwired: 1 in, 4 out]
            n139 = call <vilib>:"Close Config Data.vi"("error in (no error)"=w240, "write file if changed (T)"=TRUE ("write configuration file? (F)"), "refnum"=w241) -> ()  [unwired: 9 out]
            n140 = call "_Save Config File.vi"("GUI Method"=w247, "File Type (config)"=_File_Type."Diagnostic Method", "advisory dialog? (display:T)"=FALSE, "start path  (Not A Path)"=w248) -> ()  [unwired: 4 in, 4 out]
            n141 = global write "_Global Configuration.vi" "Run"(FALSE ("Update")) -> ()
            n142 = event-data("Discard?"=w259) -> ()  [unwired: 1 in, 1 out]
          }
          event Timeout {
            n143 = event-data() -> ()  [unwired: 4 out]
            n144 = Unbundle By Name(w262) -> ("Update"=w261:bool, "Running"=w260:bool)
            n145 = case shown="False" w261 {
              tunnel: w262 -> [w266 w310]
              tunnel: [w265 w308] -> w264
              tunnel: w260 -> [w268 _]
              tunnel: w263 -> [w267 _]
              frame False {
                n146 = case shown="True" w268 {
                  tunnel: w267 -> [_ w275]
                  tunnel: w266 -> [w269 w271]
                  tunnel: [w269 w270] -> w265
                  frame False {
                  }
                  frame True {
                    n147 = Dequeue Element(queue=w275, timeout in ms (-1)=1) -> (element=w273:cluster{T7, dbl, "error out":errorcluster}, timed out?=w272:bool)  [unwired: 1 in, 2 out]
                    n148 = case shown="True" w272 {
                      tunnel: w273 -> [w281 _]
                      tunnel: w271 -> [w277 w298]
                      tunnel: [w276 w298] -> w270
                      frame False {
                        n149 = Unbundle(w281) -> (w280:T7, w278:dbl, "error out"=w279:errorcluster)
                        n150 = case shown="\"End\"" w280 {
                          tunnel: w279 -> [_ w287 w291]
                          tunnel: w278 -> [_ _ _]
                          tunnel: w277 -> [w282 w286 w290]
                          tunnel: [w282 w285 w290] -> w276
                          frame "Init", Default {
                          }
                          frame "End" {
                            w288 = u8 0 ("Disabled")
                            n151 = property on="Run" class="Bool"("Visible"=TRUE) -> ()  [unwired: 2 in, 2 out]
                            n152 = property on="Cancel" class="Bool"("Visible"=FALSE) -> ()  [unwired: 2 in, 2 out]
                            n153 = call "_Handle Error.vi"("error in (no error)"=w287) -> ()  [unwired: 2 in, 5 out]
                            n154 = property on="Acquire" class="Bool (strict)"("Disabled"=w288) -> ()  [unwired: 2 in, 2 out]
                            n155 = property on="MCA" class="Bool (strict)"("Disabled"=w288) -> ()  [unwired: 2 in, 2 out]
                            n156 = property on="Scan#" class="DigNum (strict)"("Disabled"=w288) -> ()  [unwired: 2 in, 2 out]
                            n157 = Bundle By Name(cluster=w286, "Running"=FALSE) -> (w285:T17)
                          }
                          frame "Error" {
                            n158 = call "_Handle Error.vi"("error in (no error)"=w291) -> ()  [unwired: 2 in, 5 out]
                          }
                        }
                      }
                      frame True {
                        n159 = call "_Current Data Global.vi"("Operation"=_Data_Operation."Get Data") -> ("Latest Raw Data"=w294:i32[], "CurrentData"=w293:T18[])  [unwired: 3 in, 2 out]
                        n160 = global write "_Global Configuration.vi" "Spectrum"(w294) -> ()
                        n161 = call "_Update Display Property 2.vi"("Spectrum in"=w294) -> ()  [unwired: 7 out]
                        n162 = Index Array(array=w293) -> (element=w292:T18)  [unwired: 1 in]
                        n163 = Unbundle By Name(w292) -> ("Scan#"=w296:i32, "Run Time (mS)"=w295:i32)
                        n164 = local write "Run Time"(w295) -> ()
                        n165 = local write "Scan#"(w296) -> ()
                      }
                    }
                  }
                }
              }
              frame True {
                n166 = Unbundle By Name(w310) -> ("Method.Unit"=w307:bool, "Method"=w311:T2)
                n167 = property on="BloUpdate" class="Bool (strict)"("Value (Signaling)"=TRUE) -> ()  [unwired: 2 in, 2 out]
                n168 = Bundle("Scan Type"="Scan Type", "Unit"=w307, "Count1"="Count1", "Count2"="Count2", "Time1"="Time1", "Time2"="Time2", "Scans"="Scans", "Step Size"="Step Size", "Lens Table"="Lens Table") -> (w319:T21)  [unwired: 1 out]
                n169 = call "_Validate Lens Property.vi"("Lens Property In"=w319, "Method In"=w311) -> ("Lens Table"=w313:string[][], "Lens Property Out"=w318:T22, "Method Out"=w305:T2)  [unwired: 2 in, 2 out]
                n170 = Unbundle By Name(w318) -> ("Scan Type"=w312:u8, "Unit"=w306:bool, "Count1"=w316:dbl, "Count2"=w315:dbl, "Time1"=w299:dbl, "Time2"=w300:dbl, "Scans"=w314:i32, "Step Size"=w317:dbl, "Start DAC"=→"DAC Value":i32, "Ramp Time (ms)"=→"Run Time":i32)
                n171 = property on="Lens Table" class="MCListbox (strict)"("Item Names"=w313) -> ()  [unwired: 2 in, 2 out]
                n172 = local write "Method"(w305) -> ()
                n173 = Bundle By Name(cluster=w310, "Method"=w305, "Update"=FALSE) -> (w308:T17)
                n174 = local write "Scan Type"(w312) -> ()
                n175 = local write "Unit"(w306) -> ()
                n176 = local write "Count1"(w316) -> ()
                n177 = local write "Count2"(w315) -> ()
                n178 = local write "Time1"(w299) -> ()
                n179 = local write "Time2"(w300) -> ()
                n180 = local write "Scans"(w314) -> ()
                n181 = local write "Step Size"(w317) -> ()
              }
            }
          }
          event "Lens Table": Value Change {
            n182 = event-data() -> ("NewVal"=w343:i32)  [unwired: 1 out]
            n183 = Unbundle By Name(w338) -> ("Method.Unit"=w327:bool, "Method.Lenses"=w339:T3[])
            n184 = Array Size(array=w339) -> (size(s)=w340:i32)
            n185 = Decrement(x=w340) -> (x-1=w341:i32)
            n186 = In Range and Coerce(upper limit=w341, x=w343, lower limit=0) -> (coerced(x)=w334:i32)  [unwired: 1 out]
            n187 = local write "Lens Table"(w334) -> ()
            n188 = Index Array(array=w339, index=w334) -> (element=w337:T3)
            n189 = Index Array(array=w335, index=w334) -> (element=w330:T9)
            n190 = Unbundle By Name(w337) -> ("Scan Type"=w336:u8, "Value 1"=w347:dbl, "Value 2"=w346:dbl, "Time 1"=w345:dbl, "Time 2"=w351:dbl, "Scans"=w350:i32, "Step Size"=w348:dbl)
            n191 = Unbundle By Name(w330) -> ("Ch#"=w333:u8, "Slope"=w332:dbl, "Offset"=w331:dbl)
            n192 = local write "Time1"(w345) -> ()
            n193 = local write "Time2"(w351) -> ()
            n194 = local write "Scans"(w350) -> ()
            n195 = property on="Scan Type" class="Ring (strict)"("Value (Signaling)"=w336) -> ()  [unwired: 2 in, 2 out]
            n196 = case shown="False" w327 {
              selector: w327 -> [_ w376]
              tunnel: w348 -> [w357 w372]
              tunnel: w346 -> [w358 w373]
              tunnel: w347 -> [w355 w375]
              tunnel: [w355 w379] -> w328
              tunnel: [w358 w378] -> w349
              tunnel: [w357 w377] -> w329
              tunnel: [w354 w371] -> w344
              tunnel: w333 -> [w356 _]
              tunnel: w332 -> [w353 _]
              tunnel: w331 -> [w352 _]
              tunnel: w330 -> [_ w370]
              frame False {
                n197 = case shown="1, 4" w356 {
                  tunnel: w355 -> [w362 w365 w368]
                  tunnel: [w359 w364 w367] -> w354
                  tunnel: w353 -> [w361 _ _]
                  tunnel: w352 -> [w360 _ _]
                  frame Default {
                    n198 = Multiply(x=w362, y=w361) -> (x*y=w363:dbl)
                    n199 = Add(x=w363, y=w360) -> (x+y=w359:dbl)
                  }
                  frame 1, 4 {
                    n200 = global read "_Global Configuration.vi" "Calibration"() -> (w366:dbl[][])
                    n201 = call "_Convert Mass to DAC.vi"("Calibration Table"=w366, "Mass"=w365) -> ("DAC Value"=w364:dbl)  [unwired: 2 in, 3 out]
                  }
                  frame 2, 5 {
                    n202 = global read "_Global Configuration.vi" "Calibration 2"() -> (w369:dbl[][])
                    n203 = call "_Convert Mass to DAC.vi"("Calibration Table"=w369, "Mass"=w368) -> ("DAC Value"=w367:dbl)  [unwired: 2 in, 3 out]
                  }
                }
              }
              frame True {
                # "Convert to DAC units"
                n204 = Bundle(w376, "Value 1"=w375, "Value 2"=w373, "Step Size"=w372) -> (w374:T23)  [unwired: 1 out]
                n205 = call "_Switch Lens Property Unit.vi"("Lens Property In"=w374, "Configuration"=w370) -> ("DAC Value"=w371:i32, "Step Size"=w377:dbl, "Count2"=w378:dbl, "Count1"=w379:dbl)  [unwired: 1 in, 1 out]
              }
            }
            n206 = local write "DAC Value"(w344) -> ()
            n207 = local write "Count1"(w328) -> ()
            n208 = local write "Count2"(w349) -> ()
            n209 = local write "Step Size"(w329) -> ()
          }
          event "Scan Type": Value Change {
            n210 = event-data() -> ("NewVal"=w392:u8)  [unwired: 6 out]
            n211 = case shown="1" w392 {
              tunnel: ["Lens Value" "Low Value" "Start Value"] -> w391
              tunnel: ["High Value" "High Value" "Stop Value"] -> w390
              tunnel: ["Low Dwell (ms)" "Low Time (ms)" "Dwell Time (ms)"] -> w389
              tunnel: ["High Dwell (ms)" "High Time (ms)" "Pause Time (ms)"] -> w388
              tunnel: [w397 w402 w404] -> w387
              tunnel: [w397 w402 w404] -> w386
              tunnel: [w397 w402 w404] -> w385
              tunnel: [w397 w402 w404] -> w384
              tunnel: [w397 FALSE w404] -> w383
              frame 0, Default {
                w397 = FALSE
                # "For Single"
              }
              frame 1 {
                w402 = TRUE
                # "For Dual"
              }
              frame 2 {
                w404 = TRUE
                # "For Ramp"
              }
            }
            n212 = property on="Count2" class="DigNum (strict)"("Visible"=w387) -> ()  [unwired: 2 in, 2 out]
            n213 = property on="Time1" class="DigNum (strict)"("Visible"=w386) -> ()  [unwired: 2 in, 2 out]
            n214 = property on="Time2" class="DigNum (strict)"("Visible"=w385) -> ()  [unwired: 2 in, 2 out]
            n215 = property on="Scans" class="DigNum (strict)"("Visible"=w384) -> ()  [unwired: 2 in, 2 out]
            n216 = property on="Step Size" class="DigNum (strict)"("Visible"=w383) -> ()  [unwired: 2 in, 2 out]
            n217 = property on="Count1" class="DigNum (strict)"("Caption.Text"=w391) -> ()  [unwired: 2 in, 2 out]
            n218 = property on="Count2" class="DigNum (strict)"("Caption.Text"=w390) -> ()  [unwired: 2 in, 2 out]
            n219 = property on="Time1" class="DigNum (strict)"("Caption.Text"=w389) -> ()  [unwired: 2 in, 2 out]
            n220 = property on="Time2" class="DigNum (strict)"("Caption.Text"=w388) -> ()  [unwired: 2 in, 2 out]
            n221 = Bundle By Name(cluster=w382, "Update"=TRUE) -> (w381:T17)
          }
          event "Run": Value Change {
            n222 = event-data() -> ()  [unwired: 7 out]
            n223 = stacked-sequence {
              tunnel: w414 -> [_ _ _ w438 _ _]
              tunnel: w413 -> [w418 _ _ _ _ _]
              tunnel: w412 -> [_ _ w423 _ _ _]
              tunnel: [_ _ w422 _ _ _] -> w410
              frame #0 {
                w416 = u8 1 ("Disabled")
                n224 = Flush Queue(queue=w418) -> ()  [unwired: 1 in, 3 out]
                n225 = call <vilib>:"Set Busy.vi"() -> ()  [unwired: 4 in, 8 out]
                n226 = property on="Scan#" class="DigNum (strict)"("Disabled"=w416) -> ()  [unwired: 2 in, 2 out]
                n227 = property on="Acquire" class="Bool (strict)"("Disabled"=w416) -> ()  [unwired: 2 in, 2 out]
                n228 = property on="MCA" class="Bool (strict)"("Disabled"=w416) -> ()  [unwired: 2 in, 2 out]
                n229 = property on="Run" class="Bool"("Visible"=FALSE) -> ()  [unwired: 2 in, 2 out]
                n230 = property on="Cancel" class="Bool"("Visible"=TRUE) -> ()  [unwired: 2 in, 2 out]
              }
              frame #1 {
                n231 = Wait (ms)(milliseconds to wait=u32 180) -> ()  [unwired: 1 out]
              }
              frame #2 {
                w420 = T24 0 items=["Diagnostics", "Tune", "Acquisition"] ("RunModule")
                n232 = case shown="True" "Acquire" {
                  tunnel: w423 -> [w425 w430]
                  tunnel: [w425 w427] -> w422
                  frame False {
                  }
                  frame True {
                    n233 = local read "Data File:"() -> (w431:path)
                    n234 = call "_Get File.vi"("Start Path"=w431) -> ("Seleted File"=w432:path, "Succeeded"=w428:bool)  [unwired: 5 in, 2 out]
                    n235 = local write "Acquire"(w428) -> ()
                    n236 = case shown="True" w428 {
                      tunnel: w432 -> [_ w434]
                      tunnel: w431 -> [w433 _]
                      tunnel: [w433 w434] -> w429
                      frame False {
                      }
                      frame True {
                        n237 = local write "Data File:"(w434) -> ()
                      }
                    }
                    n238 = Bundle By Name(cluster=w430, "Method.Data Path"=w429, "Method.Acquire"=w428) -> (w427:T17)
                    n239 = Unbundle By Name(w427) -> ("Method"=w426:T2)
                    n240 = local write "Method"(w426) -> ()
                  }
                }
                n241 = global write "_Global Configuration.vi" "Run"(TRUE ("Update")) -> ()
                n242 = global write "_Global Configuration.vi" "RunModule"(w420) -> ()
              }
              frame #3 {
                n243 = local read "Scan Type"() -> (w437:u8)
                n244 = Equal?(x=w437, y=u16 1) -> (x = y?=w435:bool)
                n245 = case shown="True" w435 {
                  selector: w435 -> [_ w443]
                  tunnel: w438 -> [w441 _]
                  frame False {
                    w440 = FALSE ("Wait until done")
                    n246 = invoke class="VI" method="Run VI"(reference=w441, "Wait until done"=w440, "Auto Dispose Ref"=w440) -> ()  [unwired: 2 in, 5 out]
                    n247 = local write "Scan#"(u32 0 ("Scan#")) -> ()
                  }
                  frame True {
                    n248 = local write "Dual Run"(w443) -> ()
                    n249 = property on="Dual Run" class="Bool (strict)"("Visible"=w443) -> ()  [unwired: 2 in, 2 out]
                    n250 = call "_Remote Run Dual.vi"() -> ("error out"=w442:errorcluster)  [unwired: 2 in, 5 out]
                    n251 = call "_Handle Error.vi"("error in (no error)"=w442) -> ()  [unwired: 2 in, 5 out]
                  }
                }
              }
              frame #4 {
                n252 = Wait (ms)(milliseconds to wait=u32 800) -> ()  [unwired: 1 out]
              }
              frame #5 {
                n253 = call <vilib>:"Unset Busy.vi"() -> ()  [unwired: 2 in, 10 out]
              }
            }
            n254 = Bundle By Name(cluster=w410, "Running"=TRUE) -> (w409:T17)
          }
          event "Cancel": Value Change {
            n255 = event-data() -> ()  [unwired: 7 out]
            n256 = stacked-sequence {
              tunnel: w447 -> [_ w451 _]
              tunnel: [_ w450 _] -> w446
              tunnel: w445 -> [_ w449 _]
              frame #0 {
                n257 = call <vilib>:"Set Busy.vi"() -> ()  [unwired: 4 in, 8 out]
                n258 = global write "_Global Configuration.vi" "Run"(FALSE ("Update")) -> ()
              }
              frame #1 {
                n259 = local read "Dual Run"() -> (w452:bool)
                n260 = case shown="True" w452 {
                  tunnel: w451 -> [w454 w464]
                  tunnel: [w454 w463] -> w450
                  tunnel: w449 -> [w453 _]
                  frame False {
                    n261 = while {
                      tunnel: w453 -> [w459]
                      stop <- w456 stop-if-true
                      n262 = property class="VI"(reference=w459) -> ("Exec.State"=w458:T15)  [unwired: 1 in, 2 out]
                      n263 = Wait (ms)(milliseconds to wait=u32 180) -> ()  [unwired: 1 out]
                      n264 = Equal?(x=w458, y=T15."Idle") -> (x = y?=w456:bool)
                    }
                  }
                  frame True {
                    w465 = u8 0 ("Disabled")
                    w462 = FALSE
                    n265 = property on="Run" class="Bool"("Visible"=TRUE) -> ()  [unwired: 2 in, 2 out]
                    n266 = property on="Cancel" class="Bool"("Visible"=FALSE) -> ()  [unwired: 2 in, 2 out]
                    n267 = local write "Dual Run"(w462) -> ()
                    n268 = property on="Dual Run" class="Bool (strict)"("Visible"=w462) -> ()  [unwired: 2 in, 2 out]
                    n269 = property on="Acquire" class="Bool (strict)"("Disabled"=w465) -> ()  [unwired: 2 in, 2 out]
                    n270 = property on="MCA" class="Bool (strict)"("Disabled"=w465) -> ()  [unwired: 2 in, 2 out]
                    n271 = property on="Scan#" class="DigNum (strict)"("Disabled"=w465) -> ()  [unwired: 2 in, 2 out]
                    n272 = Bundle By Name(cluster=w464, "Running"=w462) -> (w463:T17)
                    n273 = call "_Remote Communicate.vi"("Command"=_RT_Command."Stop") -> ()  [unwired: 5 in, 4 out]
                  }
                }
              }
              frame #2 {
                n274 = call "_Remote Wait Until Done.vi"() -> ("error out"=w467:errorcluster)  [unwired: 2 in, 1 out]
                n275 = call <vilib>:"Unset Busy.vi"() -> ()  [unwired: 2 in, 10 out]
                n276 = call "_Remote Park Lens.vi"("error in"=w467) -> ()  [unwired: 1 in, 6 out]
              }
            }
          }
          event "BloUpdate": Value Change {
            n277 = event-data() -> ()  [unwired: 7 out]
            n278 = Unbundle By Name(w469) -> ("Running"=w468:bool)
            n279 = local write "BloUpdate"(FALSE) -> ()
            n280 = stacked-sequence {
              seq-local: [_ w473 _ _] -> [_ _ _ w474]
              tunnel: w468 -> [_ w472 _ _]
              frame #0 {
                n281 = call <vilib>:"Set Busy.vi"() -> ()  [unwired: 4 in, 8 out]
              }
              frame #1 {
                n282 = call "_Remote BlockUpdate.vi"("Filter (T)"=FALSE, "Running"=w472) -> ("error out"=w473:errorcluster)  [unwired: 1 in, 4 out]
              }
              frame #2 {
                n283 = call <vilib>:"Unset Busy.vi"() -> ()  [unwired: 2 in, 10 out]
              }
              frame #3 {
                n284 = call "_Handle Error.vi"("error in (no error)"=w474) -> ()  [unwired: 2 in, 5 out]
              }
            }
          }
          event "NewMethod": Value Change {
            n285 = event-data() -> ()  [unwired: 2 out]
            n286 = local write "NewMethod"(FALSE) -> ()
            n287 = Unbundle By Name(w482) -> ("Running"=w476:bool, "Method"=w484:T2)
            n288 = property on="Lens Table" class="MCListbox (strict)"("Value (Signaling)"=0) -> ()  [unwired: 2 in, 2 out]
            n289 = Unbundle By Name(w484) -> ("Q3DC EN"=w479:bool, "Run Mode"=w478:T1, "Acquire"=w495:bool, "MCA"=w494:bool, "Q1DC EN"=w498:bool, "Q1 POL"=w497:bool, "Q3 POL"=w496:bool, "Averaging"=w490:bool, "Log Scale"=w491:bool, "CPS"=w492:bool, "Data Path"=w493:path, "Lenses"=w486:T3[])  [unwired: 1 out]
            n290 = Array Size(array=w486) -> (size(s)=w488:i32)
            n291 = Array Size(array=w485) -> (size(s)=w489:i32)
            n292 = Not Equal?(x=w488, y=w489) -> (x != y?=w487:bool)
            n293 = case shown="True" w487 {
              tunnel: w485 -> [_ w503]
              tunnel: [w500 w501] -> w483
              tunnel: w486 -> [w500 _]
              frame False {
              }
              frame True {
                n294 = for {
                  tunnel: w503 -> [w506] mode=indexing
                  tunnel: T3 {"Scan Type"=0, "Scans"=1, "Time 1"=1.0, "Time 2"=1.0, "Value 1"=0.0, "Value 2"=0.0, "Step Size"=1.0} ("Lenses") -> [w507]
                  tunnel: [w504] -> w501 mode=indexing
                  n295 = Unbundle By Name(w506) -> ("Def+"=w505:dbl)
                  n296 = Bundle By Name(cluster=w507, "Value 1"=w505, "Value 2"=w505) -> (w504:T3)
                }
              }
            }
            n297 = stacked-sequence {
              tunnel: w498 -> [w512 _ _]
              tunnel: w497 -> [w510 _ _]
              tunnel: w496 -> [w511 _ _]
              tunnel: w495 -> [_ _ w532]
              tunnel: w494 -> [_ _ w531]
              tunnel: w493 -> [_ w526 _]
              tunnel: w492 -> [_ w525 _]
              tunnel: w491 -> [_ w524 _]
              tunnel: w490 -> [_ w523 _]
              tunnel: w479 -> [w513 _ _]
              tunnel: w478 -> [_ _ w530]
              tunnel: w476 -> [w508 _ _]
              frame #0 {
                n298 = local write "Q2DC EN"(w513) -> ()
                n299 = local write "Q1DC EN"(w512) -> ()
                n300 = local write "Q1 POL"(w510) -> ()
                n301 = local write "Q2 POL"(w511) -> ()
                n302 = Number To Boolean Array(number=u16 0) -> (Boolean array=w519:bool[])
                n303 = Replace Array Subset(array=w519, new element #1=w510, index #1=0 ("index"), new element #2=w511, index #2=1 ("index"), new element #3=w512, index #3=2 ("index"), new element #4=w513, index #4=3 ("index")) -> (w514:bool[])
                n304 = Boolean Array To Number(Boolean array=w514) -> (number=w509:u16)
                n305 = case shown="False" w508 {
                  tunnel: w509 -> [w521 _]
                  frame False {
                    n306 = call "_Remote Communicate.vi"("DC Param"=w521, "Command"=_RT_Command."Set Pol and DC") -> ()  [unwired: 4 in, 4 out]
                  }
                  frame True {
                  }
                }
              }
              frame #1 {
                n307 = local write "Averaging"(w523) -> ()
                n308 = local write "Log Scale"(w524) -> ()
                n309 = local write "CPS"(w525) -> ()
                n310 = call "_Read Spectrum File.vi"("advisory dialog? (display:T)"=FALSE, "start path  (Not A Path)"=w526) -> ("new file path"=→"Data File:":path, "Scan# out"=w527:u32)  [unwired: 1 in, 5 out]
                n311 = local write "Scan#"(w527) -> ()
              }
              frame #2 {
                n312 = local write "Acquire"(w532) -> ()
                n313 = local write "MCA"(w531) -> ()
                n314 = global read "_Global Configuration.vi" "Spectrum"() -> (w533:i32[])
                n315 = property on="Run Mode" class="Enum (strict)"("Val(Sgnl)"=w530) -> ()  [unwired: 2 in, 2 out]
                n316 = call "_Update Display Property 2.vi"("Spectrum in"=w533) -> ()  [unwired: 7 out]
              }
            }
            n317 = Bundle By Name(cluster=w482, "Method.Negative"=FALSE, "Method.Mass Ranges"=T4[] [], "Method.Lenses"=w483) -> (w481:T17)
          }
          event "Swtich Polarity": Value Change {
            n318 = event-data() -> ()  [unwired: 7 out]
            n319 = Unbundle By Name(w536) -> ("Method.Lenses"=w534:T3[], "Running"=w535:bool)
            n320 = case shown="False" w535 {
              tunnel: w536 -> [w543 w549]
              tunnel: [w541 w549] -> w537
              tunnel: w534 -> [w539 _]
              frame False {
                n321 = local read "Lens Table"() -> (w544:i32)
                n322 = local read "Count1"() -> (w548:dbl)
                n323 = local read "Count2"() -> (w547:dbl)
                n324 = call "_Switch Polarity.vi"("Lenses"=w539, "Start Value"=w548, "Stop Value"=w547, "index"=w544, "Unit"="Unit") -> ("Lenses 2"=w542:T3[], "Start Value 2"=w546:dbl, "Stop Value 2"=w545:dbl)  [unwired: 1 in]
                n325 = local write "Count1"(w546) -> ()
                n326 = local write "Count2"(w545) -> ()
                n327 = Bundle By Name(cluster=w543, "Method.Lenses"=w542, "Update"=TRUE) -> (w541:T17)
              }
              frame True {
                n328 = One Button Dialog(message="You must wait until the run is finish before you can switch lens polarity.") -> ()  [unwired: 2 out]
              }
            }
          }
          event "Q1DC EN", "Q1 POL", "Q2 POL", "Q2DC EN": Value Change {
            n329 = event-data() -> ()  [unwired: 2 out]
            n330 = Number To Boolean Array(number=u16 0) -> (Boolean array=w563:bool[])
            n331 = Replace Array Subset(array=w563, new element #1="Q1 POL", index #1=0 ("index"), new element #2="Q2 POL", index #2=1 ("index"), new element #3="Q1DC EN", index #3=2 ("index"), new element #4="Q2DC EN", index #4=3 ("index")) -> (w554:bool[])
            n332 = Unbundle By Name(w552) -> ("Running"=w551:bool)
            n333 = Bundle By Name(cluster=w552, "Method.Q1DC EN"="Q1DC EN", "Method.Q1 POL"="Q1 POL", "Method.Q3 POL"="Q2 POL", "Method.Q3DC EN"="Q2DC EN") -> (w565:T17)
            n334 = Boolean Array To Number(Boolean array=w554) -> (number=w553:u16)
            n335 = case shown="False" w551 {
              tunnel: w553 -> [w568 _]
              frame False {
                n336 = call "_Remote Communicate.vi"("DC Param"=w568, "Command"=_RT_Command."Set Pol and DC") -> ("error out"=w569:errorcluster)  [unwired: 4 in, 3 out]
                n337 = property on="BloUpdate" class="Bool (strict)"("Value (Signaling)"=TRUE) -> ()  [unwired: 2 in, 2 out]
                n338 = call "_Handle Error.vi"("error in (no error)"=w569) -> ()  [unwired: 2 in, 5 out]
              }
              frame True {
              }
            }
            n339 = Unbundle By Name(w565) -> ("Method"=w566:T2)
            n340 = local write "Method"(w566) -> ()
          }
          event "CPS", "Averaging", "Log Scale": Value Change {
            n341 = event-data() -> ()  [unwired: 7 out]
            n342 = stacked-sequence {
              tunnel: w572 -> [w578 w580]
              tunnel: [w574 _] -> w571
              frame #0 {
                n343 = Bundle By Name(cluster=w578, "Method.Averaging"="Averaging", "Method.Log Scale"="Log Scale", "Method.CPS"="CPS") -> (w574:T17)
                n344 = Unbundle By Name(w574) -> ("Method"=w573:T2)
                n345 = local write "Method"(w573) -> ()
              }
              frame #1 {
                n346 = Unbundle By Name(w580) -> ("Running"=w579:bool)
                n347 = case shown="False" w579 {
                  frame False {
                    n348 = global read "_Global Configuration.vi" "Spectrum"() -> (w581:i32[])
                    n349 = call "_Update Display Property 2.vi"("Spectrum in"=w581) -> ()  [unwired: 7 out]
                  }
                  frame True {
                  }
                }
              }
            }
          }
          event "Acquire", "MCA": Value Change {
            n350 = event-data() -> ()  [unwired: 7 out]
            n351 = local read "Acquire"() -> (w585:bool)
            n352 = Bundle By Name(cluster=w586, "Method.Acquire"=w585, "Method.MCA"="MCA") -> (w582:T17)
            n353 = Unbundle By Name(w582) -> ("Method"=w583:T2)
            n354 = local write "Method"(w583) -> ()
          }
          event "Scan#": Value Change {
            n355 = event-data() -> ("NewVal"=w591:u32)  [unwired: 1 out]
            n356 = Unbundle By Name(w588) -> ("Running"=w587:bool)
            n357 = global read "_Global Configuration.vi" "# of Scans"() -> (w590:i32)
            n358 = In Range and Coerce(upper limit=w590, x=w591, lower limit=u32 1) -> (coerced(x)=w589:u32)  [unwired: 1 out]
            n359 = case shown="False" w587 {
              tunnel: w589 -> [w595 _]
              frame False {
                n360 = local read "Data File:"() -> (w597:path)
                n361 = call "_Read Spectrum File.vi"("advisory dialog? (display:T)"=FALSE, "Scan#"=w595, "start path  (Not A Path)"=w597) -> ("error"=w599:bool, "TIC"=w598:u32, "error out"=w593:errorcluster, "Scan# out"=w596:u32)  [unwired: 3 out]
                n362 = case shown="False" w599 {
                  tunnel: w598 -> [_ _]
                  tunnel: w596 -> [w601 _]
                  tunnel: w593 -> [_ w602]
                  frame False {
                    n363 = global read "_Global Configuration.vi" "Spectrum"() -> (w600:i32[])
                    n364 = local write "Scan#"(w601) -> ()
                    n365 = call "_Update Display Property 2.vi"("Spectrum in"=w600) -> ()  [unwired: 7 out]
                  }
                  frame True {
                    n366 = call "_Handle Error.vi"("error in (no error)"=w602) -> ()  [unwired: 2 in, 5 out]
                  }
                }
              }
              frame True {
                n367 = One Button Dialog(message="You must wait until the run is finish before you can load another spectrum.") -> ()  [unwired: 2 out]
              }
            }
          }
          event "Count1", "Count2", "Time1", "Time2", "Scans", "Step Size": Value Change {
            n368 = event-data() -> ()  [unwired: 2 out]
            n369 = Bundle By Name(cluster=w605, "Update"=TRUE) -> (w604:T17)
          }
          event "Unit": Value Change {
            n370 = event-data() -> ("NewVal"=w607:bool)  [unwired: 1 out]
            n371 = local read "Lens Table"() -> (w612:i32)
            n372 = local read "Step Size"() -> (w620:dbl)
            n373 = local read "Count1"() -> (w619:dbl)
            n374 = local read "Count2"() -> (w618:dbl)
            n375 = Index Array(array=w613, index=w612) -> (element=w611:T9)
            n376 = Bundle("NewVal"=w607, "Count1"=w619, "Count2"=w618, "Step Size"=w620) -> (w617:T25)  [unwired: 1 out]
            n377 = call "_Switch Lens Property Unit.vi"("Lens Property In"=w617, "Configuration"=w611) -> ("Step Size"=w614:dbl, "Count2"=w615:dbl, "Count1"=w616:dbl)  [unwired: 1 in, 2 out]
            n378 = local write "Count1"(w616) -> ()
            n379 = local write "Count2"(w615) -> ()
            n380 = local write "Step Size"(w614) -> ()
            n381 = Bundle By Name(cluster=w609, "Method.Unit"=w607, "Update"=TRUE) -> (w608:T17)
          }
          event Value Change {
            n382 = event-data() -> ("NewVal"=w622:T1)  [unwired: 1 out]
            n383 = Bundle By Name(cluster=w623, "Method.Run Mode"=w622) -> (w621:T17)
          }
        }
      }
    }
    frame #2 {
      n384 = property class="VI"(reference=w625, error in=w624, "Front Panel Window:Open"=TRUE) -> (reference out=w626:refnum<vi>, error out=w627:errorcluster)
      n385 = Close Reference(reference=w629) -> ()  [unwired: 1 in, 1 out]
      n386 = Release Queue(queue=w630) -> ()  [unwired: 1 in, 4 out]
      n387 = Close Reference(reference=w626, error in (no error)=w627) -> ()  [unwired: 1 out]
    }
  }
